vi "FoodBox.vi"(8 "Pellet in holder":bool, 9 "Active":bool=TRUE, 10 "Max pellets":u32=2, 11 "ITI":u32=500) -> (2 "Number pellets":u32=500)   [LabVIEW 2021]
uses:
  <vilib>/DAQmx/read.llb/DAQmx Read (Digital Bool 1Line 1Point).vi
  <vilib>/DAQmx/write.llb/DAQmx Write (Digital Bool 1Line 1Point).vi
  <vilib>/DAQmx/create/channels.llb/DAQmx Create Channel (DI-Digital Input).vi
  <vilib>/DAQmx/create/channels.llb/DAQmx Create Channel (DO-Digital Output).vi
  <vilib>/DAQmx/miscellaneous.llb/DAQmx Fill In Error Info.vi
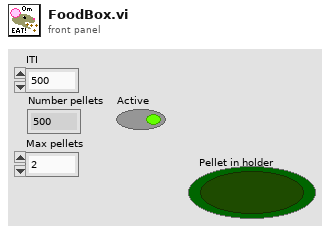
[diagram p1: front panel]
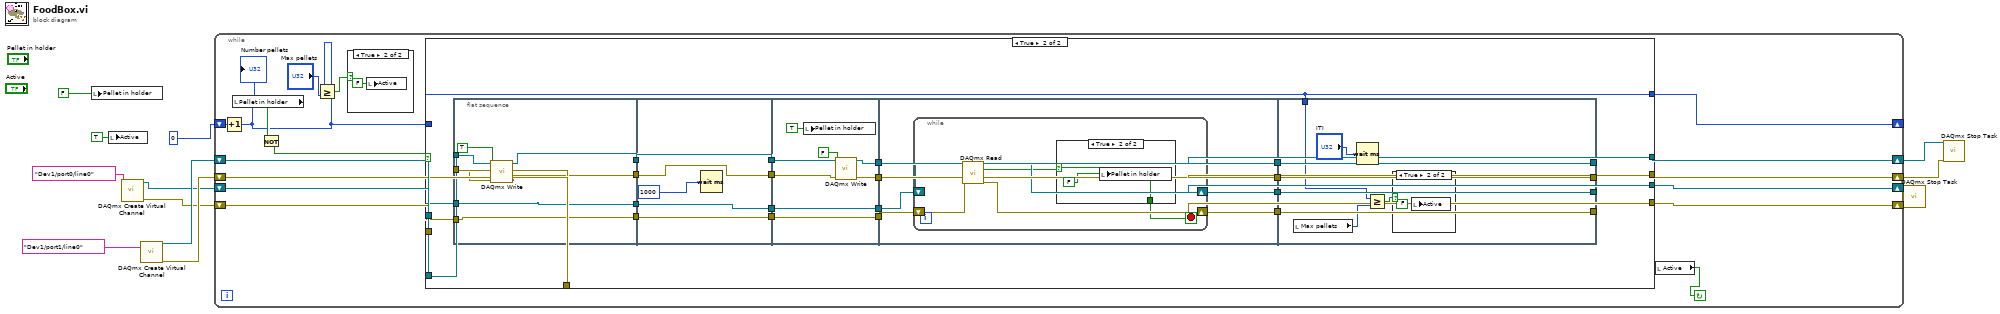
[diagram p0: block diagram]
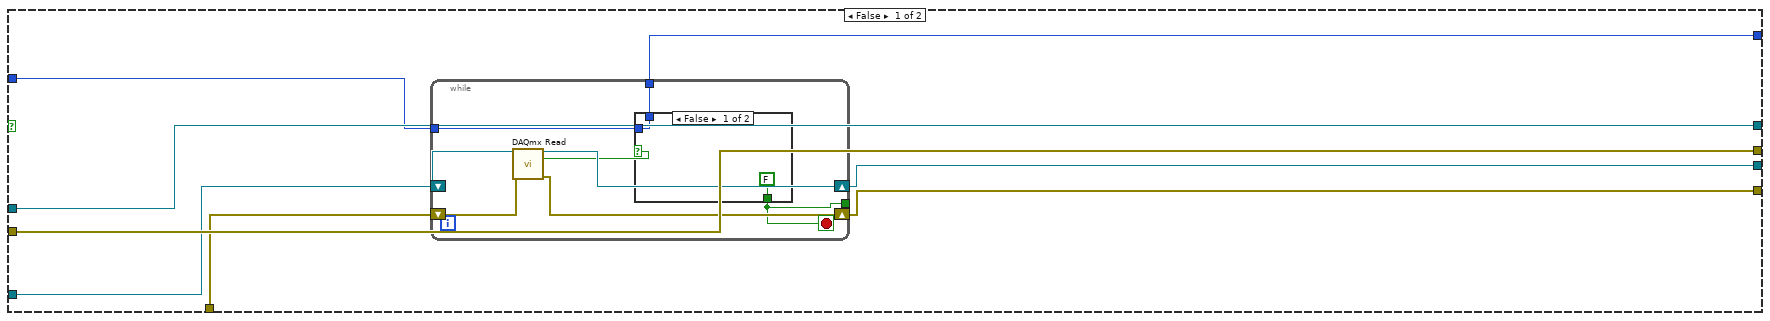
[diagram p3: hidden frame]
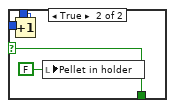
[diagram p4: hidden frame]
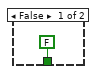
[diagram p5: hidden frame]
diagram:
  n1 = local write "Pellet in holder"(FALSE ("Pellet in holder")) -> ()
  n2 = local write "Active"(TRUE ("Active")) -> ()
  n3 = call-poly <vilib>:"DAQmx Create Virtual Channel.vi"("lines"=tag "Dev1/port0/line0") -> ("task out"=w11:refnum<k21>, "error out"=w10:errorcluster)  [unwired: 13 in]
  n4 = call-poly <vilib>:"DAQmx Create Virtual Channel.vi"("lines"=tag "Dev1/port1/line0") -> ("task out"=w13:refnum<k21>, "error out"=w12:errorcluster)  [unwired: 13 in]
  n5 = while {
    shift-right: [w22] -> w5
    shift-left: w13 -> [w28]
    shift-right: [w21] -> w4
    shift-left: w12 -> [w27]
    shift-right: [w24] -> w9
    shift-left: w11 -> [w26]
    shift-right: [w23] -> w8
    shift-left: w10 -> [w25]
    shift-right: [w19] -> _
    shift-left: u32 0 ("Number pellets") -> [w18]
    stop <- w17 continue-if-true
    n6 = Increment(x=w18) -> (x+1=w14:u32)
    "Number pellets" <- w14
    n7 = local read "Pellet in holder"() -> (w20:bool)
    n8 = Not(x=w20) -> (.not. x?=w29:bool)
    n9 = Greater Or Equal?(x=w14, y="Max pellets") -> (x >= y?=w16:bool)
    n10 = case shown="True" w16 {
      frame False {
      }
      frame True {
        n11 = local write "Active"(FALSE ("Active")) -> ()
      }
    }
    n12 = case shown="True" w29 {
      tunnel: [w38 w73] -> w22
      tunnel: [w37 w72] -> w21
      tunnel: w28 -> [w35 w69]
      tunnel: w27 -> [w36 w68]
      tunnel: w26 -> [w38 w66]
      tunnel: w25 -> [w37 w63]
      tunnel: [w33 w59] -> w24
      tunnel: [w34 w58] -> w23
      tunnel: w14 -> [w32 w53]
      tunnel: [w31 w53] -> w19
      frame False {
        n13 = while {
          shift-right: [w43] -> w33
          shift-left: w35 -> [w46]
          shift-right: [w44] -> w34
          shift-left: w36 -> [w45]
          tunnel: [w41] -> _
          tunnel: w32 -> [w40]
          tunnel: [w39] -> w31
          stop <- w41 stop-if-true
          n14 = call-poly <vilib>:"DAQmx Read.vi"("task/channels in"=w46, "error in"=w45) -> ("task out"=w43:refnum<k21>, "data"=w42:bool, "error out"=w44:errorcluster)  [unwired: 11 in]
          n15 = case shown="False" w42 {
            selector: w42 -> [_ w52]
            tunnel: [FALSE w52] -> w41
            tunnel: w40 -> [w47 w50]
            tunnel: [w47 w49] -> w39
            frame False {
            }
            frame True {
              n16 = Increment(x=w50) -> (x+1=w49:u32)
              n17 = local write "Pellet in holder"(FALSE ("Pellet in holder")) -> ()
            }
          }
        }
      }
      frame True {
        n18 = flat-sequence {
          tunnel: [w83] -> w77
          tunnel: [w82] -> w76
          tunnel: w69 -> [w81]
          tunnel: w68 -> [w80]
          tunnel: [w79] -> w67
          tunnel: w66 -> [w79]
          tunnel: w63 -> [w78]
          tunnel: [w78] -> w60
          tunnel: [w89] -> w75
          tunnel: w77 -> [w89]
          tunnel: [w88] -> w74
          tunnel: w76 -> [w88]
          tunnel: w67 -> [w87]
          tunnel: [w87] -> w64
          tunnel: [w86] -> w61
          tunnel: w60 -> [w86]
          tunnel: w75 -> [w96]
          tunnel: w74 -> [w95]
          tunnel: [w94] -> w71
          tunnel: [w93] -> w70
          tunnel: [w92] -> w65
          tunnel: w64 -> [w92]
          tunnel: [w91] -> w62
          tunnel: w61 -> [w91]
          tunnel: w71 -> [w103]
          tunnel: w70 -> [w102]
          tunnel: w65 -> [w101]
          tunnel: w62 -> [w100]
          tunnel: [w103] -> w57
          tunnel: [w102] -> w56
          tunnel: [w99] -> w55
          tunnel: [w98] -> w54
          tunnel: [w117] -> w59
          tunnel: [w118] -> w58
          tunnel: [w119] -> w72
          tunnel: [w120] -> w73
          tunnel: w57 -> [w120]
          tunnel: w56 -> [w119]
          tunnel: w55 -> [w118]
          tunnel: w54 -> [w117]
          tunnel: w53 -> [w114]
          frame #0 {
            n19 = call-poly <vilib>:"DAQmx Write.vi"("task/channels in"=w81, "data"=TRUE, "error in"=w80) -> ("task out"=w83:refnum<k21>, "error out"=w82:errorcluster)  [unwired: 10 in, 1 out]
          }
          frame #1 {
            n20 = Wait (ms)(milliseconds to wait=u32 1000) -> ()  [unwired: 1 out]
          }
          frame #2 {
            n21 = local write "Pellet in holder"(TRUE ("Pellet in holder")) -> ()
            n22 = call-poly <vilib>:"DAQmx Write.vi"("task/channels in"=w96, "data"=FALSE, "error in"=w95) -> ("task out"=w94:refnum<k21>, "error out"=w93:errorcluster)  [unwired: 10 in, 1 out]
          }
          frame #3 {
            n23 = while {
              shift-right: [w106] -> w98
              shift-left: w101 -> [w109]
              shift-right: [w107] -> w99
              shift-left: w100 -> [w108]
              stop <- w104 stop-if-true
              n24 = call-poly <vilib>:"DAQmx Read.vi"("task/channels in"=w109, "error in"=w108) -> ("task out"=w106:refnum<k21>, "data"=w105:bool, "error out"=w107:errorcluster)  [unwired: 11 in]
              n25 = case shown="True" w105 {
                selector: w105 -> [_ w112]
                tunnel: [FALSE w112] -> w104
                frame False {
                }
                frame True {
                  n26 = local write "Pellet in holder"(FALSE ("Pellet in holder")) -> ()
                }
              }
            }
          }
          frame #4 {
            n27 = local read "Max pellets"() -> (w113:u32)
            n28 = Wait (ms)(milliseconds to wait="ITI") -> ()  [unwired: 1 out]
            n29 = Greater Or Equal?(x=w114, y=w113) -> (x >= y?=w115:bool)
            n30 = case shown="True" w115 {
              frame False {
              }
              frame True {
                n31 = local write "Active"(FALSE ("Active")) -> ()
              }
            }
          }
        }
      }
    }
    n32 = local read "Active"() -> (w17:bool)
  }
  n33 = call <vilib>:"DAQmx Stop Task.vi"("task/channels in"=w9, "error in"=w8) -> ()  [unwired: 12 in, 2 out]
  n34 = call <vilib>:"DAQmx Stop Task.vi"("task/channels in"=w5, "error in"=w4) -> ()  [unwired: 12 in, 2 out]
